vi "Climber.vi"(0 "Climber Dev Ref":T1={"DeviceStatus"={"status"=FALSE, "code"=0, "source"=""}, "Type"=enum."PWM", "PWM"={"PWM Channel"=enum."Invalid", "DeadBand"={"Name"="", "maxPositivePwm"=0, "minPositivePwm"=0, "centerPwm"=0, "maxNegativePwm"=0, "minNegativePwm"=0, "angularRange"=0}}, "CAN"={"Device Number"=0, "SetOutput VI Ref"=variant(refnum<vi> refnum), "GetOutput VI Ref"=variant(refnum<vi> refnum), "Enable VI Ref"=variant(refnum<vi> refnum), "Disable VI Ref"=variant(refnum<vi> refnum), "Data"=variant}, "Invert"=FALSE}, 1 "Forward Climb":bool=TRUE, 2 "Backwards Climb":bool=TRUE, 3 "error in":errorcluster, 4 "Current Multiplier":dbl) -> (5 "Multiplier":dbl, 6 "error out":errorcluster)   [LabVIEW 2016]
uses:
  <vilib>/Rock Robotics/WPI/MotorControl/WPI_MotorControlDeviceRef.ctl
  <vilib>/Rock Robotics/WPI/MotorControl/WPI_MotorControlType.ctl
  <vilib>/Rock Robotics/SystemInterfaces/DIO/FPGA_DIOPWMChannel.ctl
  <vilib>/Rock Robotics/WPI/PWM/WPI_PWMDeadband.ctl
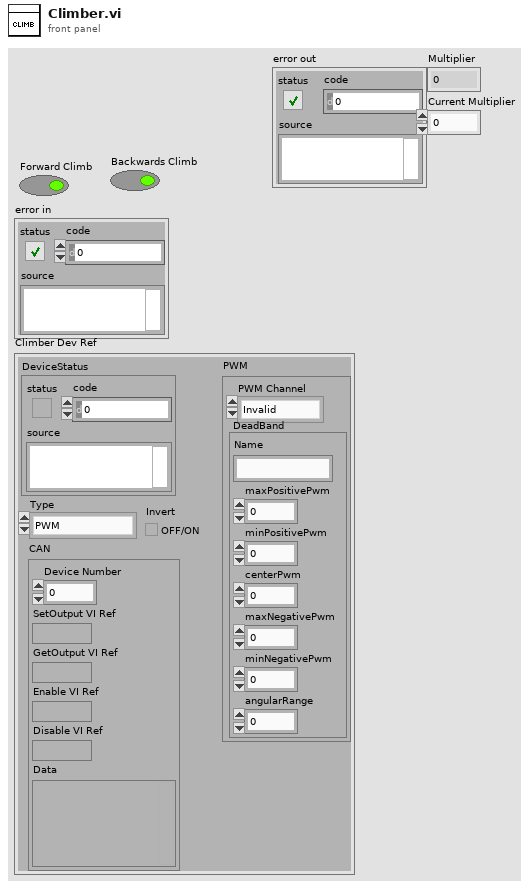
[diagram p1: front panel]
types:
  T1 = typedef "WPI_MotorControlDeviceRef.ctl" = cluster{"DeviceStatus":errorcluster, "Type":T2, "PWM":cluster{"PWM Channel":T3, "DeadBand":T4}, "CAN":cluster{"Device Number":u8, "SetOutput VI Ref":variant, "GetOutput VI Ref":variant, "Enable VI Ref":variant, "Disable VI Ref":variant, "Data":variant}, "Invert":bool}
  T2 = typedef "WPI_MotorControlType.ctl" = enum16{"PWM", "CAN"}
  T3 = typedef "FPGA_DIOPWMChannel.ctl" = enum8{"PWM 0", "PWM 1", "PWM 2", "PWM 3", "PWM 4", "PWM 5", "PWM 6", "PWM 7", "PWM 8", "PWM 9", "PWM MXP 0", "PWM MXP 1", "PWM MXP 2", "PWM MXP 3", "PWM MXP 4", "PWM MXP 5", "PWM MXP 6", "PWM MXP 7", "PWM MXP 8", "PWM MXP 9", "Invalid"}
  T4 = typedef "WPI_PWMDeadband.ctl" = cluster{"Name":string, "maxPositivePwm":i32, "minPositivePwm":i32, "centerPwm":i32, "maxNegativePwm":i32, "minNegativePwm":i32, "angularRange":u16}
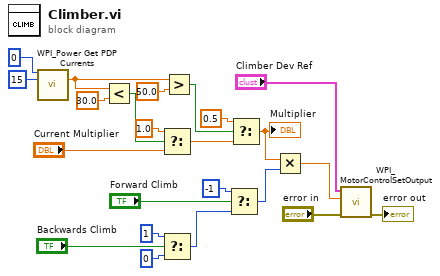
[diagram p0: block diagram]
diagram:
  n1 = call <vilib>:"WPI_Power Get PDP Currents.vi"("Power Distribution Panel (0)"=u8 0, "PDP Channel"=15) -> ("current (A)"=w2:dbl)  [unwired: 11 in, 2 out]
  n2 = Less?(x=w2, y=30.0) -> (x < y?=w8:bool)
  n3 = Select(t=1.0, s=w8, f="Current Multiplier") -> (s? t:f=w5:dbl)
  n4 = Select(t=1, s="Backwards Climb", f=0) -> (s? t:f=w17:i32)
  n5 = Greater?(x=w2, y=50.0) -> (0:w10:bool)
  n6 = Select(t=-1, s="Forward Climb", f=w17) -> (s? t:f=w4:i32)
  n7 = Select(t=0.5 ("x"), s=w10, f=w5) -> (s? t:f=w1:dbl)
  "Multiplier" <- w1
  n8 = Multiply(x=w1, y=w4) -> (x*y=w3:dbl)
  n9 = call <vilib>:"WPI_MotorControlSetOutput.vi"("error in (no error)"="error in", "Output"=w3, "MotorControlDevRef"="Climber Dev Ref") -> ("error out"=→"error out":errorcluster)  [unwired: 6 in, 2 out]
